vi "Receive String Data Only.vi"(0 "TCP Ref In":refnum<k5>, 1 "Time Out(ms)":i32=100, 2 "Re-Try":i32=5, 11 "error in (no error)":errorcluster) -> (4 "TCP Ref Out":refnum<k5>, 6 "Data":string, 15 "error out":errorcluster)   [LabVIEW 2024]
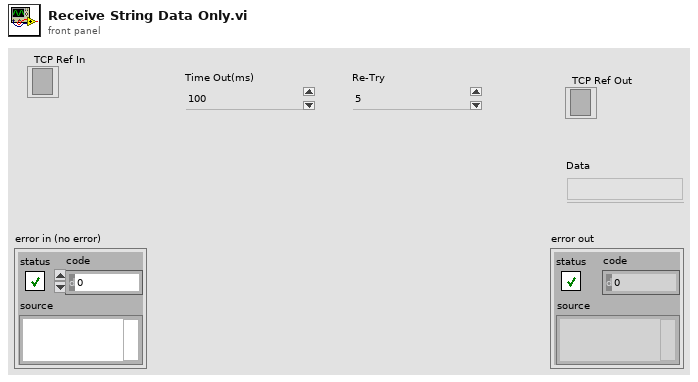
[diagram p1: front panel]
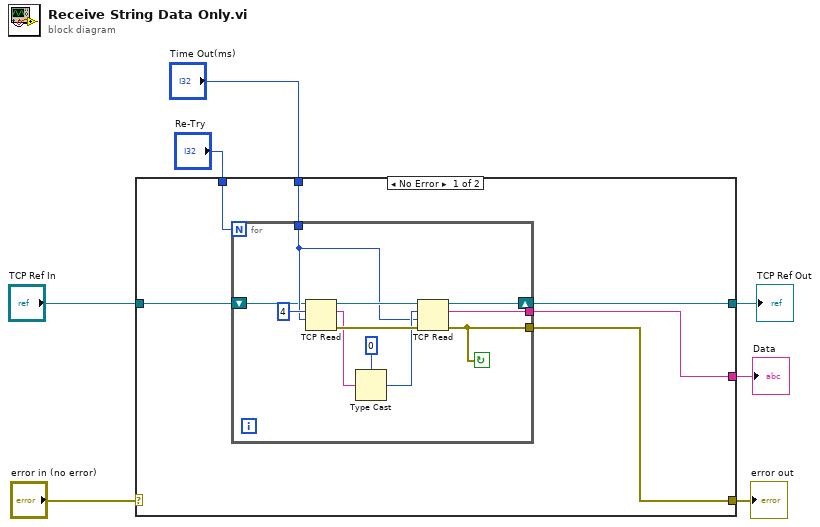
[diagram p0: block diagram]
diagram:
  n1 = case shown="No Error" "error in (no error)" {
    selector: "error in (no error)" -> [_ w26]
    tunnel: [w13 w26] -> w6
    tunnel: [w12 _] -> w5
    tunnel: "Time Out(ms)" -> [w11 _]
    tunnel: "TCP Ref In" -> [w9 w25]
    tunnel: [w10 w25] -> w2
    tunnel: "Re-Try" -> [w8 _]
    frame No Error {
      n2 = for {
        N: w8 -> [_]
        tunnel: [w14] -> w13
        tunnel: [w18] -> w12
        tunnel: w11 -> [w17]
        shift-right: [w16] -> w10
        shift-left: w9 -> [w15]
        stop <- w14 continue-if-true
        n3 = TCP Read(connection ID=w15, bytes to read=4, 9:w17) -> (connection ID out=w22:refnum<k5>, data out=w20:string, error out=w23:errorcluster)  [unwired: 2 in]
        n4 = Type Cast(type=0 ("bytes to read"), x=w20) -> (*(type *) &x=w19:i32)
        n5 = TCP Read(connection ID=w22, bytes to read=w19, error in (no error)=w23, 9:w17) -> (connection ID out=w16:refnum<k5>, data out=w18:string, error out=w14:errorcluster)  [unwired: 1 in]
      }
    }
    frame Error {
    }
  }
  "error out" <- w6
  "Data" <- w5
  "TCP Ref Out" <- w2
